vi "GetRotationMatrix2D.vi"(8 "error in":errorcluster, 9 "Scale":dbl=1.0, 10 "Angle":dbl, 11 "Point":T1) -> (0 "error out":errorcluster, 3 "Result":dbl[][](array[numeric]))   [LabVIEW 2020, in "OpenLvVision_OpenCv.lvlib"]
doc: "Calculates an affine matrix of 2D rotation."
uses:
  OpenLvVision_OpenCv.lvlib
  TypeDef/Point/2D_PointSGL.ctl
  Dlls/OlvOpenCvWrapper.dll
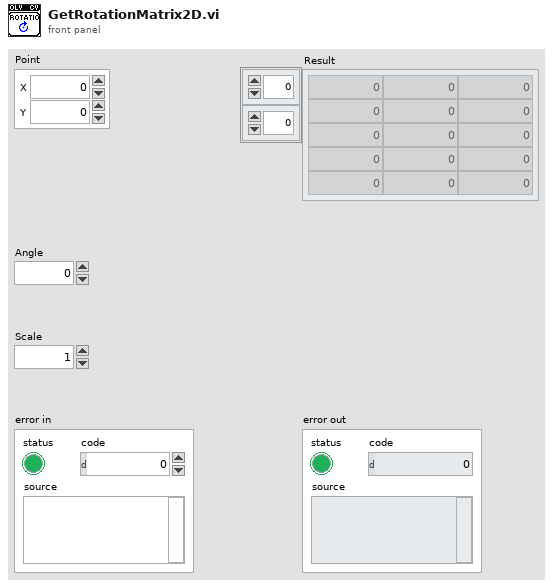
[diagram p1: front panel]
types:
  T1 = typedef "OpenLvVision_OpenCv.lvlib/2D_PointSGL.ctl" = cluster{"X":sgl, "Y":sgl}
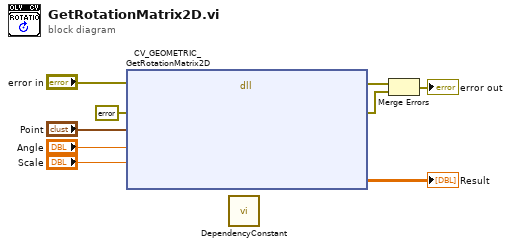
[diagram p0: block diagram]
diagram:
  n1 = dll-call lib="C:/Users/lukas/Downloads/OpenLvVision_OpenCv/SourceCode/LabView/OpenLvVision_OpenCv/Dlls/OlvOpenCvWrapper.dll" fn="CV_GEOMETRIC_GetRotationMatrix2D"(error in="error in", "Error"=errorcluster {"status"=FALSE, "code"=0, "source"=""}, "center"="Point", "angle"="Angle", "scale"="Scale") -> (error out=w7:errorcluster, "Error"=w8:errorcluster, "result"=→"Result":dbl[][])  [unwired: 7 in, 1 out]
  n2 = call "DependencyConstant.vi"() -> ()  [unwired: 12 in]
  n3 = Merge Errors(w7, w8) -> (→"error out":errorcluster)
